vi "Add Connection to State.vi"(8 "error in":errorcluster, 9 "connection":T1, 10 "state":string, 11 "routing channel in":T2 format="%.0x") -> (0 "error out":errorcluster, 3 "routing channel out":T2=18446744073709551615 format="%.0x")   [LabVIEW 2017, in "Routing and Faulting Scripting.lvlib"]
uses:
  Routing and Faulting Scripting.lvlib
  <vilib>/NI Veristand/Custom Device API/Custom Device Item Ref.ctl
  Shared/Connection.ctl
  NationalInstruments.VeriStand.SystemDefinitionAPI
  Constants/Scripting Constants.vi
  <vilib>/NI Veristand/Custom Device API/Custom Device API.lvlib
  Shared/Routing and Faulting Shared.lvlib
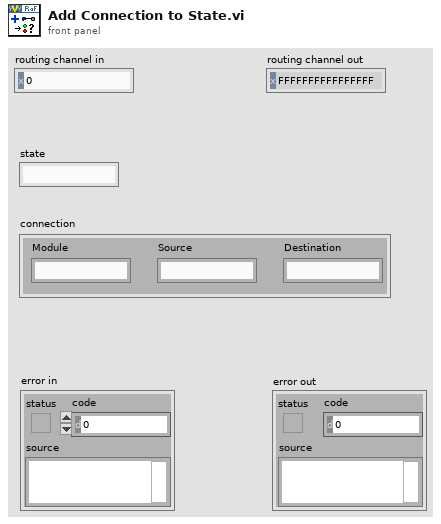
[diagram p1: front panel]
types:
  T1 = typedef "Routing and Faulting Shared.lvlib/Connection.ctl" = cluster{"Module":string, "Source":string, "Destination":string}
  T2 = typedef "Custom Device API.lvlib/Custom Device Item Ref.ctl" = u64
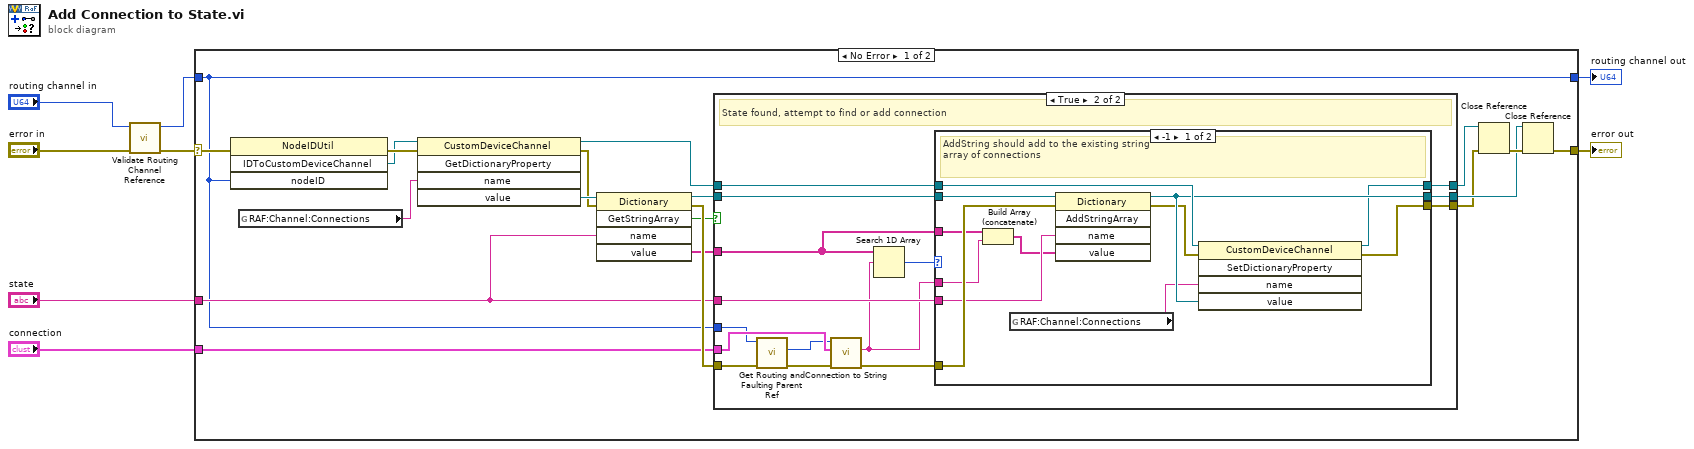
[diagram p0: block diagram]
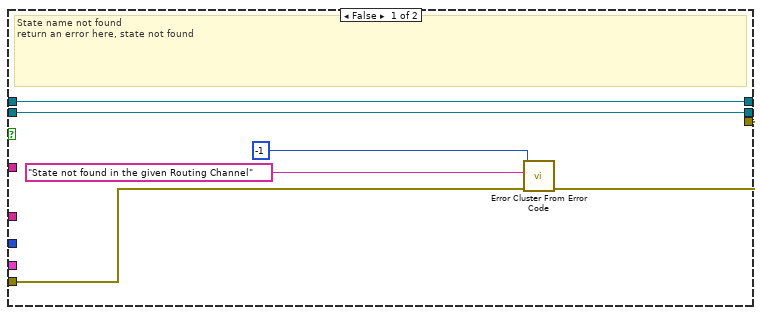
[diagram p2: hidden frame]
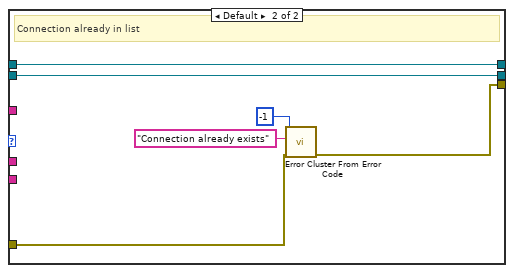
[diagram p3: hidden frame]
diagram:
  n1 = call "Validate Routing Channel Reference.vi"("error in"="error in", "routing channel in"="routing channel in") -> ("error out"=w3:errorcluster, "routing channel out"=w1:T2)  [unwired: 8 in]
  n2 = case shown="No Error" w3 {
    selector: w3 -> [w23 w68]
    tunnel: [w26 w68] -> w7
    tunnel: w1 -> [w9 w67]
    tunnel: [w9 w67] -> w6
    tunnel: "state" -> [w17 _]
    tunnel: "connection" -> [w12 _]
    frame No Error {
      n3 = invoke class="NodeIDUtil" method="IDToCustomDeviceChannel"(error in=w23, "nodeID"=w9) -> (error out=w24:errorcluster, "IDToCustomDeviceChannel"=w14:refnum<k24>)  [unwired: 2 in, 2 out]
      n4 = global read "Scripting Constants.vi" "RAF:Channel:Connections"() -> (w11:string)
      n5 = invoke class="CustomDeviceChannel" method="GetDictionaryProperty"(reference=w14, error in=w24, "name"=w11) -> (reference out=w10:refnum<k24>, error out=w20:errorcluster, "value"=w21:refnum<k24>)  [unwired: 2 in, 2 out]
      n6 = invoke class="Dictionary" method="GetStringArray"(reference=w21, error in=w20, "name"=w17) -> (reference out=w18:refnum<k24>, error out=w27:errorcluster, "GetStringArray"=w19:bool, "value"=w22:string[])  [unwired: 2 in, 1 out]
      n7 = case shown="True" w19 {
        tunnel: w22 -> [_ w41]
        tunnel: [w31 w47] -> w15
        tunnel: w17 -> [_ w46]
        tunnel: w18 -> [w30 w45]
        tunnel: [w30 w44] -> w16
        tunnel: w10 -> [w29 w43]
        tunnel: [w29 w42] -> w13
        tunnel: w12 -> [_ w40]
        tunnel: w9 -> [_ w37]
        tunnel: w27 -> [w28 w36]
        frame False {
          # "State name not found\nreturn an error here, state not found"
          n8 = call <vilib>:"Error Cluster From Error Code.vi"("error in (no error)"=w28, "error message (\"\")"="State not found in the given Routing Channel" ("error message (\"\")"), "error code (0)"=-1) -> ("error out"=w31:errorcluster)  [unwired: 6 in]
        }
        frame True {
          # "State found, attempt to find or add connection"
          n9 = call "Get Routing and Faulting Parent Ref.vi"("error in"=w36, "routing and faulting child in"=w37) -> ("error out"=w35:errorcluster, "routing and faulting"=w34:T2)  [unwired: 7 in, 1 out]
          n10 = call "Connection to String.vi"("error in"=w35, "connection"=w40, "routing and faulting in"=w34) -> ("error out"=w38:errorcluster, "string"=w39:string)  [unwired: 5 in, 2 out]
          n11 = Search 1D Array(1D array=w41, element=w39) -> (index of element=w48:i32)  [unwired: 1 in]
          n12 = case shown="-1" w48 {
            tunnel: [w54 w64] -> w47
            tunnel: w46 -> [w59 _]
            tunnel: w45 -> [w58 w63]
            tunnel: [w56 w63] -> w44
            tunnel: w43 -> [w57 w62]
            tunnel: [w53 w62] -> w42
            tunnel: w41 -> [w52 _]
            tunnel: w39 -> [w51 _]
            tunnel: w38 -> [w60 w61]
            frame -1 {
              # "AddString should add to the existing string\narray of connections"
              n13 = Build Array (concatenate)(w52, w51) -> (w50:string[])
              n14 = global read "Scripting Constants.vi" "RAF:Channel:Connections"() -> (w49:string)
              n15 = invoke class="Dictionary" method="AddStringArray"(reference=w58, error in=w60, "name"=w59, "value"=w50) -> (reference out=w56:refnum<k24>, error out=w55:errorcluster)  [unwired: 1 in, 3 out]
              n16 = invoke class="CustomDeviceChannel" method="SetDictionaryProperty"(reference=w57, error in=w55, "name"=w49, "value"=w56) -> (reference out=w53:refnum<k24>, error out=w54:errorcluster)  [unwired: 1 in, 3 out]
            }
            frame Default {
              # "Connection already in list"
              n17 = call <vilib>:"Error Cluster From Error Code.vi"("error in (no error)"=w61, "error message (\"\")"="Connection already exists" ("error message (\"\")"), "error code (0)"=-1) -> ("error out"=w64:errorcluster)  [unwired: 6 in]
            }
          }
        }
      }
      n18 = Close Reference(reference=w13, error in (no error)=w15) -> (error out=w25:errorcluster)
      n19 = Close Reference(reference=w16, error in (no error)=w25) -> (error out=w26:errorcluster)
    }
    frame Error {
    }
  }
  "routing channel out" <- w6
  "error out" <- w7
